vi "16进制输入.vi"(1 "16进制输出":string) -> (0 "正常显示":string)   [LabVIEW 2018, in "qingshan.lvlib"]
uses:
  qingshan.lvlib
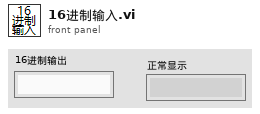
[diagram p1: front panel]
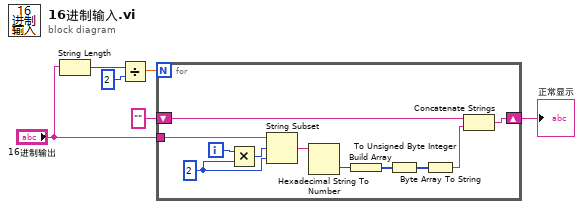
[diagram p0: block diagram]
diagram:
  n1 = String Length(string="16进制输出") -> (length=w6:i32)
  n2 = Divide(x=w6, y=2) -> (x/y=w4:dbl)
  n3 = for {
    N: w4 -> [_]
    tunnel: "16进制输出" -> [w17]
    shift-right: [w7] -> w1
    shift-left: "" -> [w8]
    i -> [w16]
    w14 = 2 ("y")
    n4 = Multiply(x=w16, y=w14) -> (x*y=w15:i32)
    n5 = String Subset(string=w17, offset (0)=w15, length (rest)=w14) -> (substring=w13:string)
    n6 = Hexadecimal String To Number ("十六进制数字符串至数值转换")(string=w13) -> (number=w12:u32)  [unwired: 2 in, 1 out]
    n7 = Build Array(w12) -> (w11:u32[])
    n8 = To Unsigned Byte Integer(number=w11) -> (unsigned 8bit integer=w10:u8[])
    n9 = Byte Array To String(unsigned byte array=w10) -> (string=w9:string)
    n10 = Concatenate Strings(w8, w9) -> (w7:string)
  }
  "正常显示" <- w1
